vi "VI Copyright.vi"() -> ()   [LabVIEW 2020, in "System Einstellungen V2.lvlib"]
uses:
  System Einstellungen V2.lvlib
  IAG-Logo-Auto B02.ctl
  Aktioen FGV System Konstanten.ctl
  Allgemein/allgemeine Sub-VIs.lvlib
panel:
  in  "IAG":T1
  out "Software-Version:":string
  out "Seriennummer:":string
  # "IAG Prüfstandstechnik G.m.b.H.\nIndustriestrasse 322 \n2722 Weikersdorf\nAUSTRIA\nwww.iag-ng.at"
  # "Copyright ©[2024] IAG Prüfstandstechnik G.m.b.H. \nAll rights reserved. \n\nThe Programm was developed with LabVIEW\n© 1986-2024 National Instruments. All rights reserved."
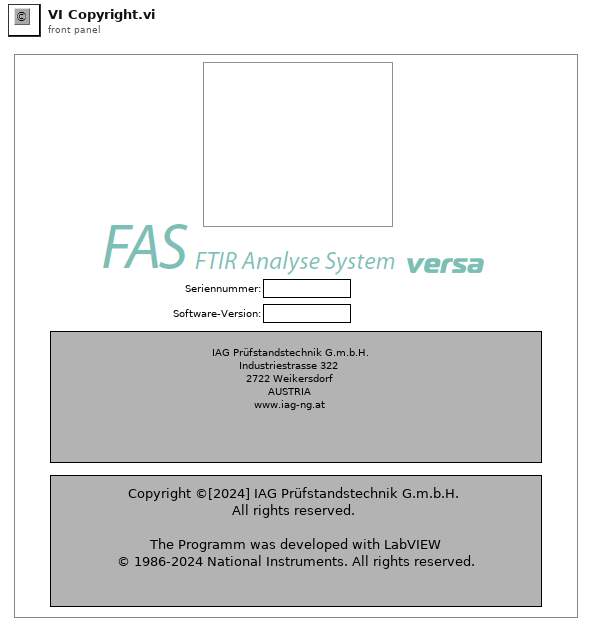
[diagram p1: front panel]
types:
  T1 = typedef "IAG-Logo-Auto B02.ctl" = bool
  T2 = typedef "System Einstellungen V2.lvlib/Aktioen FGV System Konstanten.ctl" = enum16{"lesen", "laden", "speichern", "Sprache"}
  T3 = cluster{"Modell":string, "ProjektNummer":string, "Software Version":string, "Seriennummer":string}
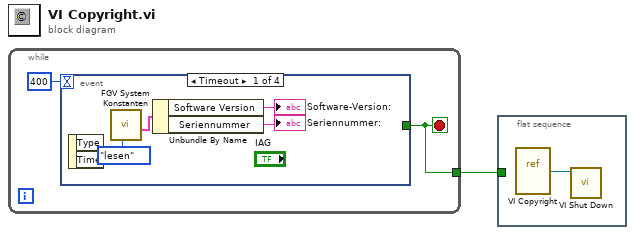
[diagram p0: block diagram]
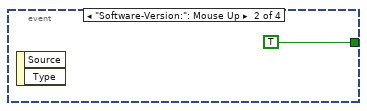
[diagram p2: hidden frame]
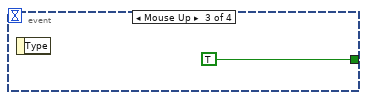
[diagram p3: hidden frame]
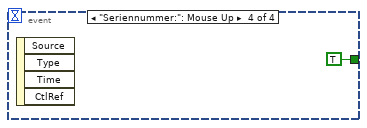
[diagram p4: hidden frame]
diagram:
  n1 = while {
    tunnel: [w2] -> w1
    stop <- w2 stop-if-true
    n2 = event shown="[0] Timeout" {
      selector: _ -> [_ _ _ _]
      dyn-events: _ -> [_ _ _ _]
      timeout: 400 -> [_ _ _ _]
      tunnel: [_ TRUE TRUE TRUE] -> w2
      event Timeout {
        n3 = event-data() -> ()  [unwired: 1 in, 2 out]
        n4 = call "FGV System Konstanten.vi"("Aktionen"=Aktioen_FGV_System_Konstanten."lesen") -> ("Cluster out"=w6:T3)  [unwired: 6 in, 4 out]
        n5 = Unbundle By Name(w6) -> ("Software Version"=→"Software-Version:":string, "Seriennummer"=→"Seriennummer:":string)
      }
      event "Software-Version:": Mouse Up {
        n6 = event-data() -> ()  [unwired: 1 in, 2 out]
      }
      event Mouse Up {
        n7 = event-data() -> ()  [unwired: 1 in, 1 out]
      }
      event "Seriennummer:": Mouse Up {
        n8 = event-data() -> ()  [unwired: 1 in, 4 out]
      }
    }
  }
  n9 = flat-sequence {
    tunnel: w1 -> [_]
    frame #0 {
      n10 = vi-ref "VI Copyright.vi"() -> (w11:refnum<vi>)
      n11 = call "VI Shut Down.vi"("VI Referenz"=w11) -> ()  [unwired: 11 in]
    }
  }
